vi "new_gain.vi"(6 "Array_in":i8[][](array[numeric])) -> ()   [LabVIEW 2010]
uses:
  glob1.vi
panel:
  out "Range":dbl[](array[numeric])
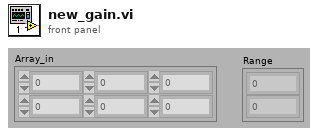
[diagram p1: front panel]
types:
  T1 = typedef "niScope vertical coupling.ctl" = i32
  T2 = cluster{"channel name":string, "input impedance":u32, "maximum input frequency":dbl, "vertical coupling":T1, "probe attenuation":dbl, "vertical range":dbl, "vertical offset":dbl, "channel enabled":bool}[]
  T3 = cluster{"channel name":string, "input impedance":u32, "maximum input frequency":dbl, "vertical coupling":T1, "probe attenuation":dbl, "vertical range":dbl, "vertical offset":dbl, "channel enabled":bool}
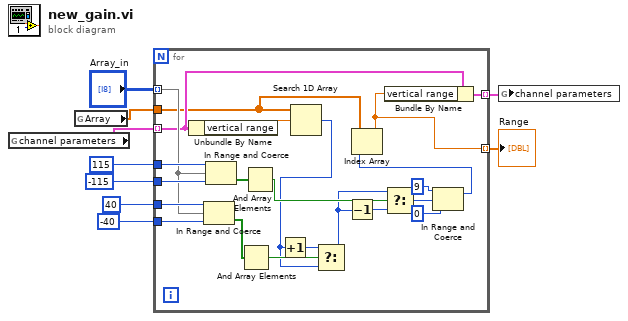
[diagram p0: block diagram]
diagram:
  n1 = global read "glob1.vi" "channel parameters"() -> (w3:T2)
  n2 = global read "glob1.vi" "Array"() -> (w4:dbl[])
  n3 = for {
    tunnel: i16 115 ("y") -> [w31]
    tunnel: i16 -115 ("y") -> [w30]
    tunnel: i16 40 ("y") -> [w29]
    tunnel: i16 -40 ("y") -> [w28]
    tunnel: "Array_in" -> [w17] mode=indexing
    tunnel: w4 -> [w13]
    tunnel: w3 -> [w14] mode=indexing
    tunnel: [w12] -> w2 mode=indexing
    tunnel: [w10] -> w1 mode=indexing
    n4 = Unbundle By Name(w14) -> ("vertical range"=w16:dbl)
    n5 = In Range and Coerce(upper limit=w29, x=w17, lower limit=w28) -> (In Range?=w25:bool[])  [unwired: 1 out]
    n6 = In Range and Coerce(upper limit=w31, x=w17, lower limit=w30) -> (In Range?=w27:bool[])  [unwired: 1 out]
    n7 = And Array Elements(Boolean array=w25) -> (logical AND=w24:bool)
    n8 = And Array Elements(Boolean array=w27) -> (logical AND=w26:bool)
    n9 = Search 1D Array(1D array=w13, element=w16) -> (index of element=w15:i32)  [unwired: 1 in]
    n10 = Increment(x=w15) -> (x+1=w23:i32)
    n11 = Select(t=w23, s=w24, f=w15) -> (s? t:f=w22:i32)
    n12 = Decrement(x=w22) -> (x-1=w21:i32)
    n13 = Select(t=w22, s=w26, f=w21) -> (s? t:f=w20:i32)
    n14 = In Range and Coerce(upper limit=9, x=w20, lower limit=0) -> (coerced(x)=w11:i32)  [unwired: 1 out]
    n15 = Index Array(array=w13, index=w11) -> (element=w10:dbl)
    n16 = Bundle By Name(cluster=w14, "vertical range"=w10) -> (w12:T3)
  }
  "Range" <- w1
  n17 = global write "glob1.vi" "channel parameters"(w2) -> ()
